vi "example_with_sub_VI.vi"() -> ()   [LabVIEW 2010]
panel:
  in  "List":i32[](array[numeric])=[0, 0, 0, 0, 0, 0, 0, 0, 0, 0]
  out "error out":errorcluster
  in  "error in":errorcluster
  out "probability not equal to 1":bool
  in  "number of unique samples":i32
  out "samples":i32[](array[numeric])
  in  "probability":dbl[](array[numeric])
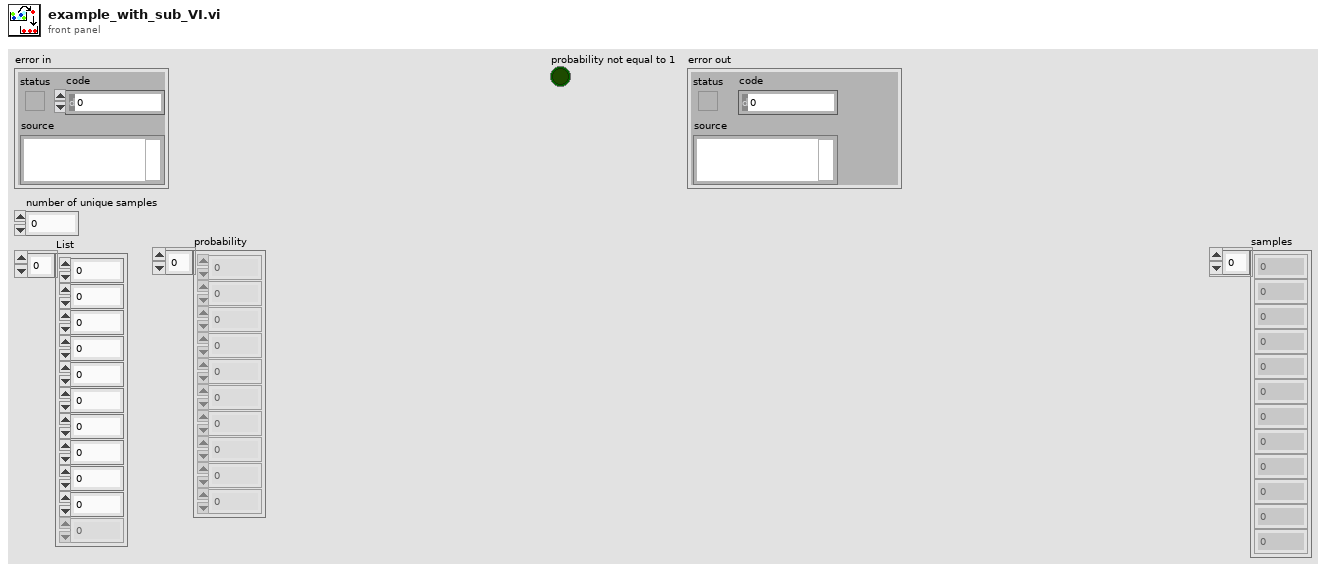
[diagram p1: front panel]
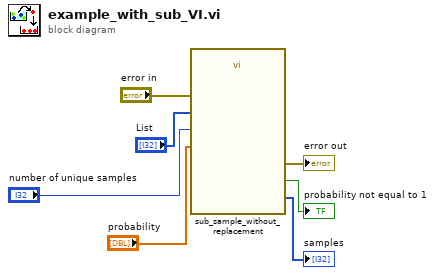
[diagram p0: block diagram]
diagram:
  n1 = call "sub_sample_without_replacement.vi"("error in (no error)"="error in", "number of unique samples"="number of unique samples", "probability"="probability", "List"="List") -> ("error out"=→"error out":errorcluster, "probability not equal to 1"=→"probability not equal to 1":bool, "unique samples"=→"samples":i32[])  [unwired: 5 in]
